vi "TelescopeHeader.vi"() -> ()   [LabVIEW 2014]
panel:
  out "Error":bool
  in  "read":bool
  in  "Exit":bool
  out "Telescope Header":string="***"
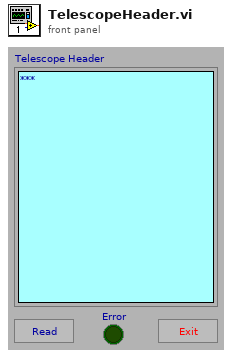
[diagram p1: front panel]
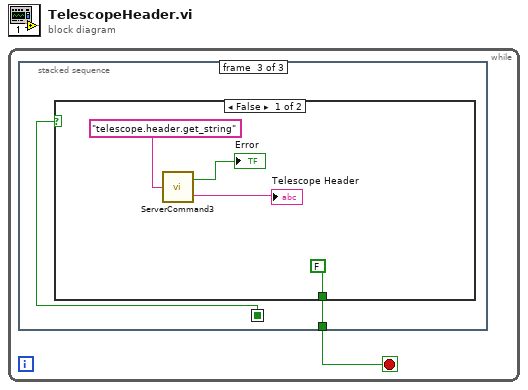
[diagram p0: block diagram]
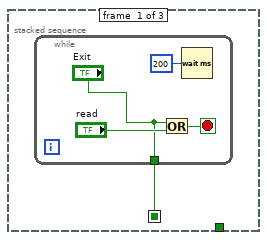
[diagram p2: hidden frame]
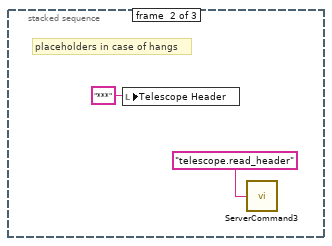
[diagram p3: hidden frame]
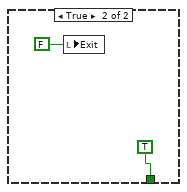
[diagram p4: hidden frame]
diagram:
  n1 = while {
    stop <- w1 stop-if-true
    n2 = stacked-sequence {
      seq-local: [w2 _ _] -> [_ _ w9]
      tunnel: [_ _ w10] -> w1
      frame #0 {
        n3 = while {
          tunnel: ["Exit"] -> w2
          stop <- w5 stop-if-true
          n4 = Or(x="Exit", y="read") -> (x .or. y?=w5:bool)
          n5 = Wait (ms)(milliseconds to wait=u32 200) -> ()  [unwired: 1 out]
        }
      }
      frame #1 {
        # "placeholders in case of hangs"
        n6 = local write "Telescope Header"("***" ("reply received")) -> ()
        n7 = call "ServerCommand3.vi"("Command"="telescope.read_header") -> ()  [unwired: 2 out]
      }
      frame #2 {
        n8 = case shown="False" w9 {
          tunnel: [FALSE TRUE] -> w10
          frame False {
            n9 = call "ServerCommand3.vi"("Command"="telescope.header.get_string") -> ("Error"=→"Error":bool, "Reply"=→"Telescope Header":string)
          }
          frame True {
            n10 = local write "Exit"(FALSE ("stop")) -> ()
          }
        }
      }
    }
  }
